vi "LabViewCode.vi"() -> ()   [LabVIEW 2013]
uses:
  <vilib>/NXT/NXT Controls/ConnectionType.ctl
  <vilib>/NXT/Subs/MotorOutput.ctl
  <vilib>/NXT/Block Support/NXT_OutputPort.ctl
  <vilib>/NXT/Dual Mode Library/Sensors/EV3_Infrared_Remote.vi
  <vilib>/NXT/NXTIO Xnodes/NXTIONodeSubVIs/LEGOMotorStatus.vi
  <vilib>/NXT/NXTIO Xnodes/NXTIONodeSubVIs/NXTMoveMotors.vi
  <vilib>/NXT/NXTIO Xnodes/AddressXNode/NXTIOAddress.xnode
  <vilib>/NXT/NXTIO Xnodes/NXTIOXNode/NXTIO.xnode
  <vilib>/NXT/Subs/LVHSConnector.ctl
  <vilib>/NXT/LegoClasses/BrickReference/BrickReference.lvclass
panel:
  in  "file path (use dialog) 2":path
  in  "file path (use dialog)":path
  out "Position 1":i32
  in  "stop":bool
  out "Numeric 3":dbl
  out "Numeric 2":dbl
  in  "actualpos":dbl
  out "Numeric":dbl
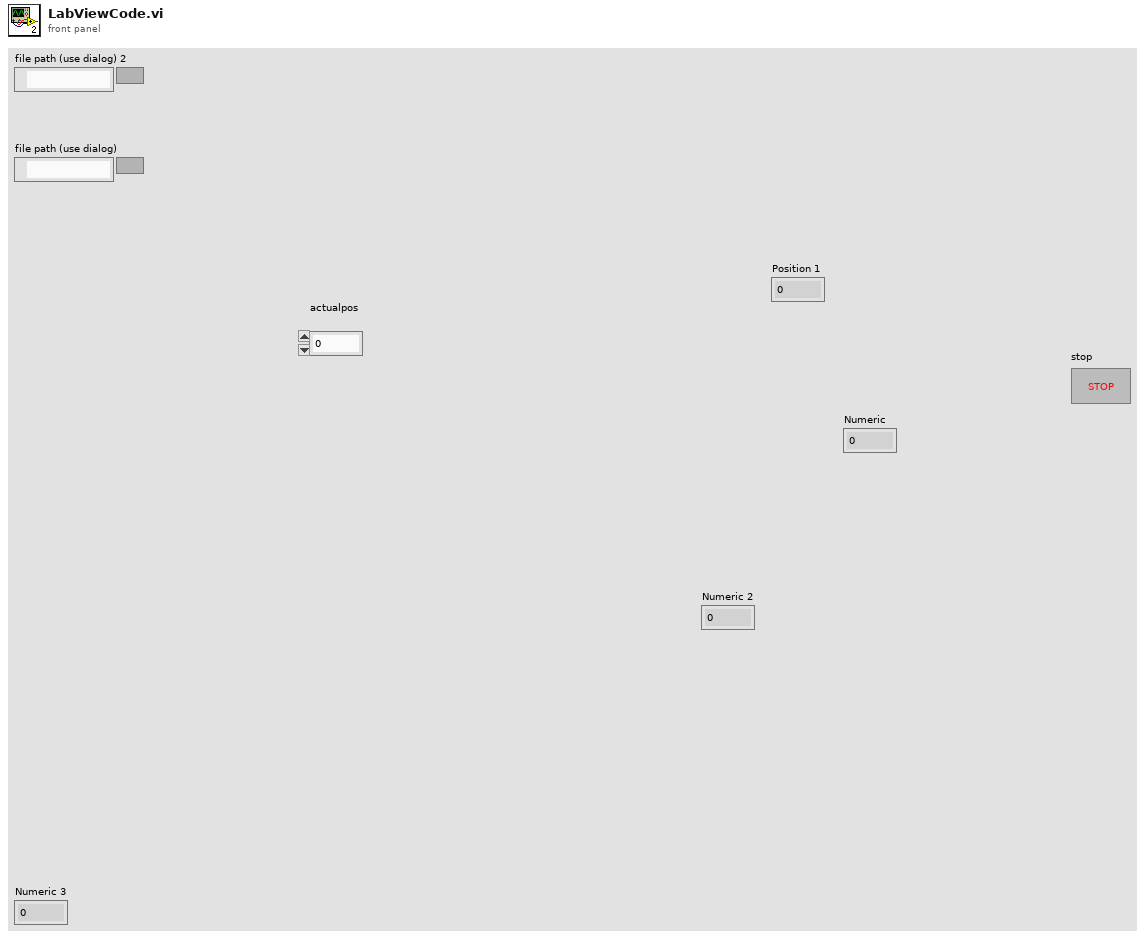
[diagram p1: front panel]
types:
  T1 = typedef "ConnectionType.ctl" = enum16{"Bluetooth", "USB", "WiFi"}
  T2 = typedef "MotorOutput.ctl" = u8
  T3 = typedef "LVHSConnector.ctl" = refnum<class "BrickReference.lvclass">
  T4 = typedef "NXT_OutputPort.ctl" = u8
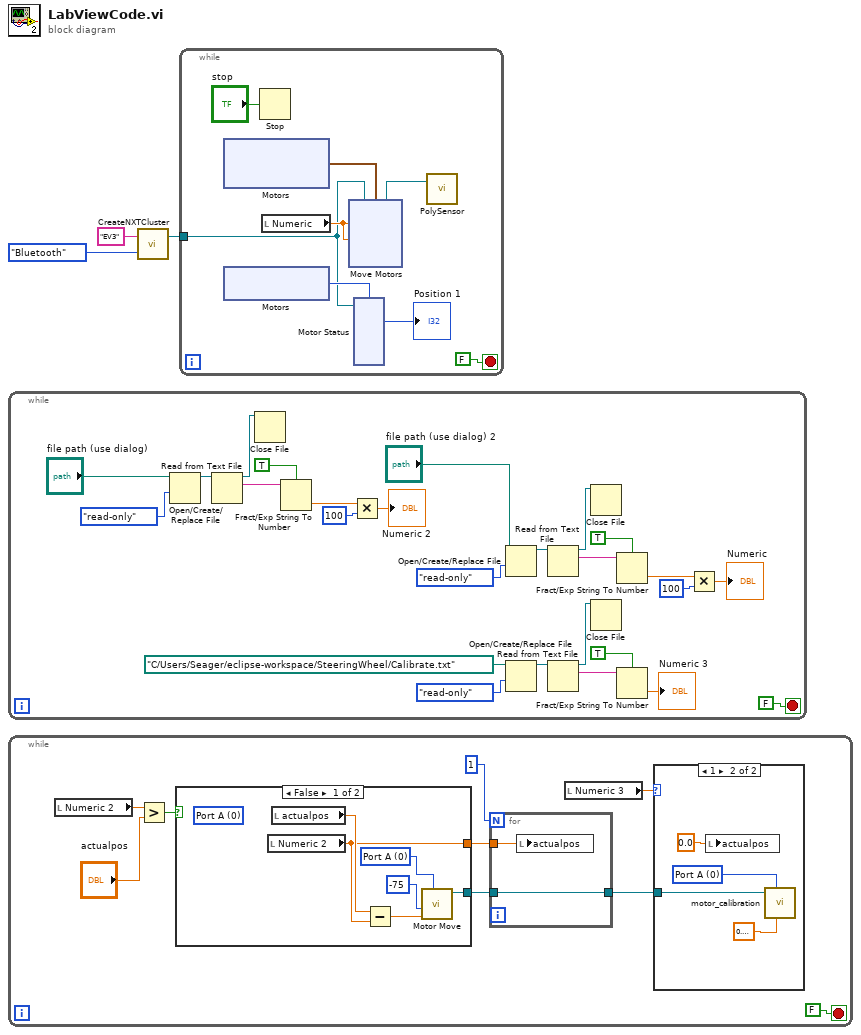
[diagram p0: block diagram]
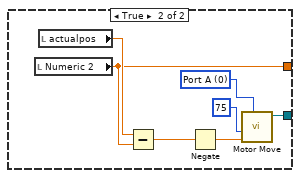
[diagram p3: hidden frame]
diagram:
  n1 = while {
    stop <- FALSE stop-if-true
    n2 = Open/Create/Replace File(file path (use dialog)="file path (use dialog)", access (0:read/write)=enum16{"read/write", "read-only", "write-only"}."read-only") -> (refnum out=w25:refnum<file>)  [unwired: 4 in, 2 out]
    n3 = Read from Text File(file (use dialog)=w25) -> (refnum out=w7:refnum<file>, text=w27:string)  [unwired: 3 in, 2 out]
    n4 = Close File(refnum=w7) -> ()  [unwired: 1 in, 2 out]
    n5 = Fract/Exp String To Number(use system decimal point (T)=TRUE, string=w27) -> (number=w29:dbl)  [unwired: 2 in, 1 out]
    n6 = Multiply(x=w29, y=100) -> (x*y=→"Numeric 2":dbl)
    n7 = Open/Create/Replace File(file path (use dialog)="file path (use dialog) 2", access (0:read/write)=enum16{"read/write", "read-only", "write-only"}."read-only") -> (refnum out=w19:refnum<file>)  [unwired: 4 in, 2 out]
    n8 = Open/Create/Replace File(file path (use dialog)=path "C:/Users/Seager/eclipse-workspace/SteeringWheel/Calibrate.txt", access (0:read/write)=enum16{"read/write", "read-only", "write-only"}."read-only") -> (refnum out=w12:refnum<file>)  [unwired: 4 in, 2 out]
    n9 = Read from Text File(file (use dialog)=w19) -> (refnum out=w8:refnum<file>, text=w17:string)  [unwired: 3 in, 2 out]
    n10 = Read from Text File(file (use dialog)=w12) -> (refnum out=w6:refnum<file>, text=w13:string)  [unwired: 3 in, 2 out]
    n11 = Close File(refnum=w8) -> ()  [unwired: 1 in, 2 out]
    n12 = Close File(refnum=w6) -> ()  [unwired: 1 in, 2 out]
    n13 = Fract/Exp String To Number(use system decimal point (T)=TRUE, string=w17) -> (number=w15:dbl)  [unwired: 2 in, 1 out]
    n14 = Fract/Exp String To Number(use system decimal point (T)=TRUE, string=w13) -> (number=→"Numeric 3":dbl)  [unwired: 2 in, 1 out]
    n15 = Multiply(x=w15, y=100) -> (x*y=→"Numeric":dbl)
  }
  n16 = while {
    stop <- FALSE stop-if-true
    n17 = local read "Numeric 2"() -> (w32:dbl)
    n18 = Greater?(x=w32, y="actualpos") -> (0:w37:bool)
    n19 = case shown="False" w37 {
      tunnel: [w46 w51] -> w35
      tunnel: [w49 w56] -> w33
      frame False {
        w45 = T2 0 items=["Port A"=0, "Port B"=1, "Port C"=2, "Ports A & B"=4, "Ports A & C"=5, "Ports B & C"=6, "All Ports"=3] ("Output Port (All Ports)")
        (unwired) T2 0 items=["Port A"=0, "Port B"=1, "Port C"=2, "Ports A & B"=4, "Ports A & C"=5, "Ports B & C"=6, "All Ports"=3] ("Output Port (All Ports)")
        n20 = local read "Numeric 2"() -> (w49:dbl)
        n21 = local read "actualpos"() -> (w50:dbl)
        n22 = Subtract(x=w50, y=w49) -> (x-y=w47:dbl)
        n23 = call "Motor Move.vi"("Output Port (All Ports)"=w45, "Angle of Rotation (360)"=w47, "Power (75)"=-75) -> ("NXT/EV3"=w46:T3)  [unwired: 8 in]
      }
      frame True {
        w54 = T2 0 items=["Port A"=0, "Port B"=1, "Port C"=2, "Ports A & B"=4, "Ports A & C"=5, "Ports B & C"=6, "All Ports"=3] ("Output Port (All Ports)")
        n24 = local read "Numeric 2"() -> (w56:dbl)
        n25 = local read "actualpos"() -> (w57:dbl)
        n26 = Subtract(x=w57, y=w56) -> (x-y=w55:dbl)
        n27 = Negate(x=w55) -> (-x=w52:dbl)
        n28 = call "Motor Move.vi"("Output Port (All Ports)"=w54, "Angle of Rotation (360)"=w52, "Power (75)"=75) -> ("NXT/EV3"=w51:T3)  [unwired: 8 in]
      }
    }
    n29 = for {
      N: 1 -> [_]
      tunnel: w35 -> [w43]
      tunnel: w33 -> [w44]
      tunnel: [w43] -> w31
      n30 = local write "actualpos"(w44) -> ()
    }
    n31 = local read "Numeric 3"() -> (w30:dbl)
    n32 = case shown="1" w30 {
      tunnel: w31 -> [_ w41]
      frame 0, Default {
      }
      frame 1 {
        w42 = T4 0 items=["Port A", "Port B", "Port C", "Port D"] ("Motors")
        n33 = local write "actualpos"(0.0 ("actualpos")) -> ()
        n34 = call "motor_calibration.vi"("NXT/EV3"=w41, "Motors"=w42, "Time (1 sec)"=sgl 0.9) -> ()  [unwired: 5 in, 1 out]
      }
    }
  }
  n35 = call <vilib>:"CreateNXTCluster.vi"("Connection Type"=ConnectionType."Bluetooth", "NXT/EV3 name"="EV3") -> ("NXT/EV3"=w1:T3)  [unwired: 2 in]
  n36 = while {
    tunnel: w1 -> [w59]
    stop <- FALSE stop-if-true
    n37 = xnode "Motors"() -> ("Motor"=w64:cluster{"Port":T4, "Port":T4})
    n38 = xnode "Motors"() -> ("Motor"=w60:T4)
    n39 = Stop(stop? (T)="stop") -> ()
    n40 = local read "Numeric"() -> (w63:dbl)
    n41 = xnode "Move Motors"("Power/Speed 2"=w63, "Power/Speed 1"=w63, "Motors"=w64, "NXT/EV3"=w59) -> ("NXT/EV3"=w62:T3)
    n42 = xnode "Motor Status"("Motors"=w60, "NXT/EV3"=w59) -> ("Position 1"=→"Position 1":i32)  [unwired: 2 out]
    n43 = call-poly <vilib>:"PolySensor.vi"("NXT/EV3"=w62) -> ()  [unwired: 2 in, 2 out]
  }
